vi "LM model function Raman positive only polybaseline.vi"(3 "output control":T1, 4 "data":T2, 5 "X":dbl[](array[numeric]) format="%#_8g", 6 "a":dbl[](array[numeric])) -> (0 "error out":errorcluster, 1 "f'(X,a)":dbl[][](array[numeric]), 2 "f(X,a)":dbl[](array[numeric]))   [LabVIEW 2015]
doc: "This template is the starting point for creating a model function to be passed to the Nonlinear Curve Fit.vi."
uses:
  <vilib>/gmath/NumericalOptimization/objective function data.ctl
  <vilib>/gmath/NumericalOptimization/LM_output select.ctl
  <vilib>/Utility/file.llb/Read From Spreadsheet File (DBL).vi
  <vilib>/gmath/NI_Gmath.lvlib
panel:
  # "Version 1.0\nAVM"
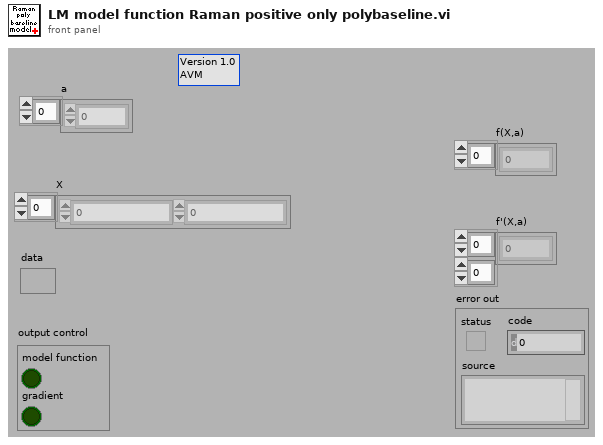
[diagram p1: front panel]
types:
  T1 = typedef "NI_Gmath.lvlib/LM_output select.ctl" = cluster{"model function":bool, "gradient":bool}
  T2 = typedef "NI_Gmath.lvlib/objective function data.ctl" = variant
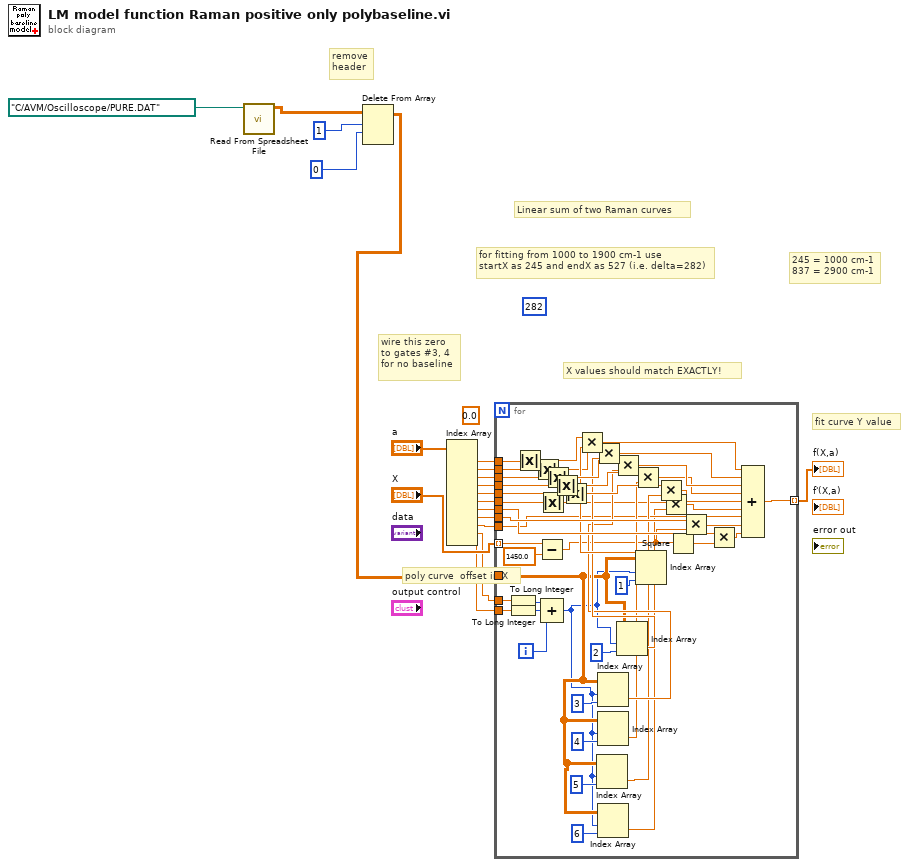
[diagram p0: block diagram]
diagram:
  (unwired) 282 ("index (row)")
  (unwired) 0.0 ("element")
  # "poly curve  offset in X"
  # "245 = 1000 cm-1\n837 = 2900 cm-1"
  # "for fitting from 1000 to 1900 cm-1 use\nstartX as 245 and endX as 527 (i.e. delta=282)"
  # "wire this zero\nto gates #3, 4\nfor no baseline"
  # "remove\nheader"
  # "X values should match EXACTLY!"
  # "Linear sum of two Raman curves"
  # "fit curve Y value"
  n1 = call-poly <vilib>:"Read From Spreadsheet File.vi"("file path (dialog if empty)"=path "C:/AVM/Oscilloscope/PURE.DAT") -> ("all rows"=w15:dbl[][])  [unwired: 6 in, 4 out]
  n2 = Delete From Array(array=w15, length=1 ("index (row)"), index (row)=0) -> (array with subset deleted=w10:dbl[][])  [unwired: 1 in, 1 out]
  n3 = Index Array(array="a") -> (element #1=w18:dbl, element #2=w17:dbl, element #3=w9:dbl, element #4=w8:dbl, element #5=w7:dbl, element #6=w1:dbl, element #7=w3:dbl, element #8=w2:dbl, element #9=w4:dbl, element #10=w6:dbl, element #11=w5:dbl)  [unwired: 11 in]
  n4 = for {
    tunnel: "X" -> [w32] mode=indexing
    tunnel: w18 -> [w63]
    tunnel: w17 -> [w34]
    tunnel: [w62] -> w16 mode=indexing
    tunnel: w10 -> [w28]
    tunnel: w9 -> [w54]
    tunnel: w8 -> [w51]
    tunnel: w6 -> [w59]
    tunnel: w5 -> [w55]
    tunnel: w2 -> [w53]
    tunnel: w3 -> [w52]
    tunnel: w7 -> [w50]
    tunnel: w4 -> [w24]
    tunnel: w1 -> [w23]
    i -> [w57]
    n5 = To Long Integer(number=w59) -> (32bit integer=w58:i32)
    n6 = To Long Integer(number=w55) -> (32bit integer=w56:i32)
    n7 = Absolute Value(x=w63) -> (abs(x)=w49:dbl)
    n8 = Absolute Value(x=w34) -> (abs(x)=w33:dbl)
    n9 = Subtract(x=w32, y=1450.0) -> (x-y=w30:dbl)
    n10 = Absolute Value(x=w23) -> (abs(x)=w22:dbl)
    n11 = Compound Arithmetic op=ADD(w58, w56, w57) -> (w27:i32)
    n12 = Absolute Value(x=w54) -> (abs(x)=w48:dbl)
    n13 = Absolute Value(x=w51) -> (abs(x)=w47:dbl)
    n14 = Absolute Value(x=w50) -> (abs(x)=w46:dbl)
    n15 = Index Array(array=w28, index (row)=w27, index (col)=5 ("index (row)")) -> (element=w40:dbl)
    n16 = Index Array(array=w28, index (row)=w27, index (col)=3 ("index (row)")) -> (element=w43:dbl)
    n17 = Index Array(array=w28, index (row)=w27, index (col)=4 ("index (row)")) -> (element=w42:dbl)
    n18 = Index Array(array=w28, index (row)=w27, index (col)=6 ("index (row)")) -> (element=w20:dbl)
    n19 = Multiply(x=w48, y=w43) -> (x*y=w37:dbl)
    n20 = Index Array(array=w28, index (row)=w27, index (col)=2 ("index (row)")) -> (element=w44:dbl)
    n21 = Multiply(x=w33, y=w44) -> (x*y=w38:dbl)
    n22 = Multiply(x=w47, y=w42) -> (x*y=w36:dbl)
    n23 = Index Array(array=w28, index (row)=w27, index (col)=1 ("index (row)")) -> (element=w45:dbl)
    n24 = Multiply(x=w49, y=w45) -> (x*y=w39:dbl)
    n25 = Multiply(x=w46, y=w40) -> (x*y=w35:dbl)
    n26 = Multiply(x=w22, y=w20) -> (x*y=w21:dbl)
    n27 = Square(x=w30) -> (x^2=w60:dbl)
    n28 = Multiply(x=w53, y=w30) -> (x*y=w25:dbl)
    n29 = Multiply(x=w52, y=w60) -> (x*y=w26:dbl)
    n30 = Compound Arithmetic op=ADD(w39, w38, w37, w36, w35, w21, w24, w25, w26) -> (w62:dbl)
  }
  "f(X,a)" <- w16
